vi "FIFOSingleChannelToHost.vi"(8 "Reset":bool, 9 "FIFO control":T1, 11 "Single Channel":T2) -> (0 "FIFO Single Channels Pixels Lost":u32, 2 "assert pixel overwritten interrupt":bool, 3 "assert FIFO overflow interrupt":bool)   [LabVIEW 2014]
uses:
  <vilib>/rvi/DataTransferAndStorage/Container/XNode/niFpgaContainer.xnode
  <vilib>/rvi/interface/RandomDataEmulation/nirviRandomDataFpgaReadWriteTemplate.vi
panel:
  # "Copyright 2014 Vidrio Technologies\nScanImage 5 software is licensed under the Apache License, Version 2.0 (the \"License\"); you may not use any files contained\nwithin the ScanImage 5 release except in compliance with the License. You may obtain a copy of the License at\n http://www.apache.org/licenses/LICENSE-2.0\nUnless required by applicable law or agreed to in writing, software distributed under the License is distributed on an\n\"AS IS\" BASIS, WITHOUT WARRANTIES OR CONDITIONS OF ANY KIND, either express or implied. See the License for the\n specific language governing permissions and limitations under the License."
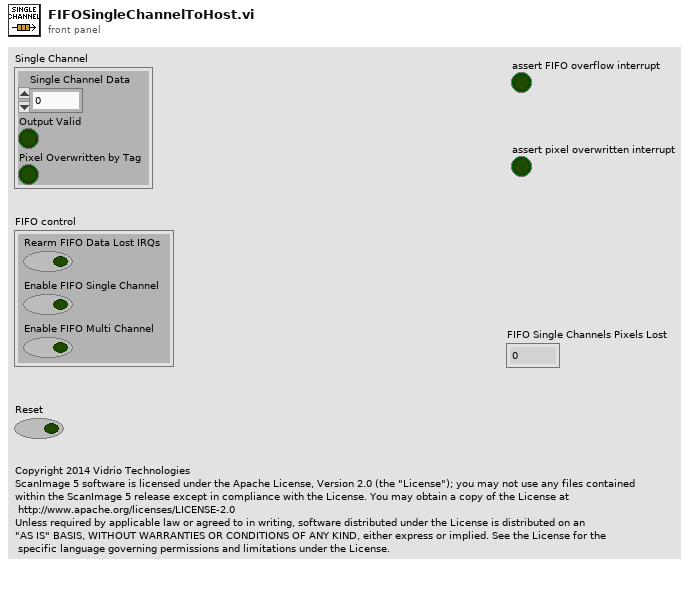
[diagram p1: front panel]
types:
  T1 = cluster{"Rearm FIFO Data Lost IRQs":bool, "Enable FIFO Single Channel":bool, "Enable FIFO Multi Channel":bool}
  T2 = cluster{"Single Channel Data":i16, "Output Valid":bool, "Pixel Overwritten by Tag":bool}
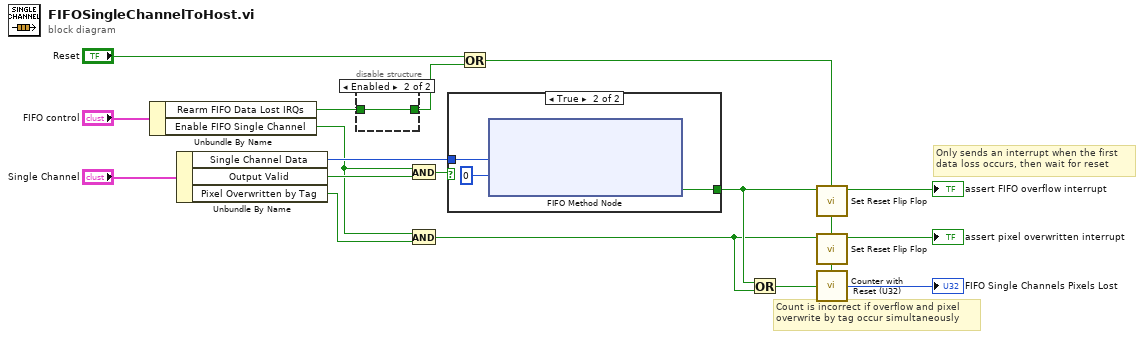
[diagram p0: block diagram]
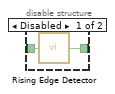
[diagram p2: hidden frame]
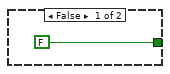
[diagram p3: hidden frame]
diagram:
  # "Count is incorrect if overflow and pixel\noverwrite by tag occur simultaneously"
  # "Only sends an interrupt when the first\ndata loss occurs, then wait for reset"
  n1 = Unbundle By Name("FIFO control") -> ("Rearm FIFO Data Lost IRQs"=w2:bool, "Enable FIFO Single Channel"=w4:bool)
  n2 = Unbundle By Name("Single Channel") -> ("Single Channel Data"=w13:i16, "Output Valid"=w10:bool, "Pixel Overwritten by Tag"=w5:bool)
  n3 = disable-structure shown="Enabled" {
    disable-tunnel: w2 -> [w19 w20]
    disable-tunnel: [w18 w20] -> w1
    frame Disabled {
      n4 = call "Rising Edge Detector.vi"("signal"=w19) -> ("edge detected"=w18:bool)  [unwired: 14 in]
    }
    frame Enabled {
    }
  }
  n5 = And(x=w4, y=w10) -> (x .and. y?=w17:bool)
  n6 = And(x=w4, y=w5) -> (x .and. y?=w3:bool)
  n7 = case shown="True" w17 {
    tunnel: [FALSE ("Timed Out?") w24] -> w7
    tunnel: w13 -> [_ w23]
    frame False {
    }
    frame True {
      n8 = xnode ("FIFO Method Node")("Element"=w23, "Timeout"=0) -> ("Timed Out?"=w24:bool)  [unwired: 1 in, 1 out]
    }
  }
  n9 = Or(x="Reset", y=w1) -> (x .or. y?=w9:bool)
  n10 = Or(x=w7, y=w3) -> (x .or. y?=w8:bool)
  n11 = call "Set Reset Flip Flop.vi"("Reset"=w9, "Set"=w7) -> ("Out"=→"assert FIFO overflow interrupt":bool)  [unwired: 9 in]
  n12 = call "Set Reset Flip Flop.vi"("Reset"=w9, "Set"=w3) -> ("Out"=→"assert pixel overwritten interrupt":bool)  [unwired: 9 in]
  n13 = call "Counter with Reset (U32).vi"("Reset?"=w9, "Increment"=w8) -> ("Counter"=→"FIFO Single Channels Pixels Lost":u32)  [unwired: 13 in]
